vi "ROI entry screen-Fit and sanity check ROIs.vi"(10 "Old ROI file's data in":dbl[][](array[numeric])=[[0.0, 0.0, 0.0, 888.0, 200.0, 60.0, 888.0, 0.0, 0.0], [0.0, 0.0, 0.0, 888.0, 250.0, 70.0, 888.0, 50.0, 10.0], [0.0, 0.0, 0.0, 0.0, 80.0, 250.0, 888.0, 20.0, 50.0]] format="%#_6f", 11 "ROI fit info":T1 {"ROI fit info"."Frame size"."Old" items=["100X100"=100, "128X128"=128, "200X200"=200, "256X256"=256, "512X512"=512, "1024x1024"=1024, "2048x2048"=2048]; "ROI fit info"."Frame size"."New" items=["100X100"=100, "128X128"=128, "200X200"=200, "256X256"=256, "512X512"=512, "1024x1024"=1024, "2048x2048"=2048]}) -> (2 "Fitted ROI data":dbl[][](array[numeric]) format="%#_6f")   [LabVIEW 2020]
uses:
  Typedefs/ROI fitting info cluster.ctl
  Typedefs/Frame Size.ctl
panel:
  out "Mismatch":bool
  out "Vertical?":bool[](array[boolean])
  out "Output OK (mismatch fixed)":bool
  # "NOTE:\nThe default values saved in the controls are used to demonstrate how a rounding error in the conversion of the second ROI is corrected by the \"Check & Correct\" module."
  # "X start"
  # "Y start"
  # "X stop"
  # "Y stop"
  # "X start"
  # "Y start"
  # "X stop"
  # "Y stop"
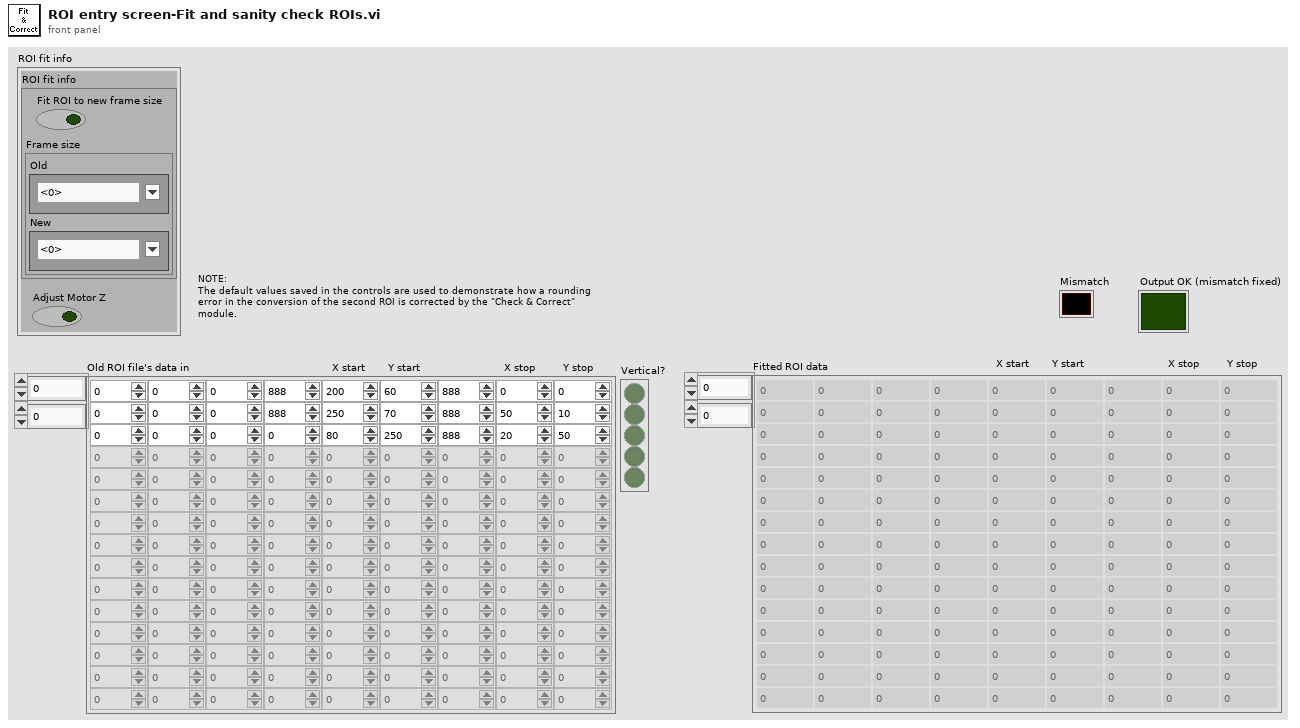
[diagram p1: front panel]
types:
  T1 = typedef "ROI fitting info cluster.ctl" = cluster{"ROI fit info":cluster{"Fit ROI to new frame size":bool, "Frame size":cluster{"Old":T2, "New":T2}}, "Adjust Motor Z":bool}
  T2 = typedef "Frame Size.ctl" = u16
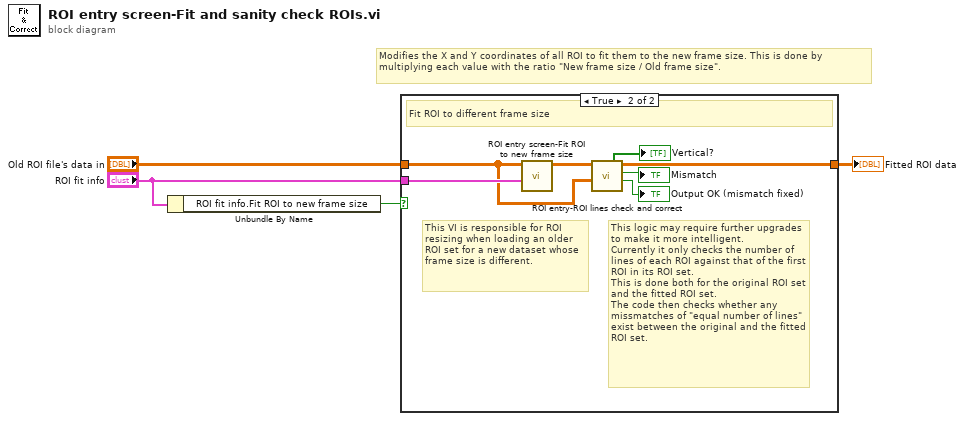
[diagram p0: block diagram]
diagram:
  # "Modifies the X and Y coordinates of all ROI to fit them to the new frame size. This is done by multiplying each value with the ratio \"New frame size / Old frame size\"."
  n1 = Unbundle By Name("ROI fit info") -> ("ROI fit info.Fit ROI to new frame size"=w4:bool)
  n2 = case shown="True" w4 {
    tunnel: "Old ROI file's data in" -> [w5 w7]
    tunnel: [w5 w11] -> w3
    tunnel: "ROI fit info" -> [_ w8]
    frame False {
      # "No need to adjust the ROI set"
    }
    frame True {
      # "This VI is responsible for ROI resizing when loading an older ROI set for a new dataset whose frame size is different."
      # "This logic may require further upgrades to make it more intelligent.\nCurrently it only checks the number of lines of each ROI against that of the first ROI in its ROI set.\nThis is done both for the original ROI set and the fitted ROI set.\nThe code then checks whether any missmatches of \"equal number of lines\" exist between the original and the fitted ROI set."
      # "Fit ROI to different frame size"
      n3 = call "ROI entry screen-Fit ROI to new frame size.vi"("ROI fit info"=w8, "Old ROI file's data in"=w7) -> ("Old ROI file's data out"=w6:dbl[][])  [unwired: 9 in]
      n4 = call "ROI entry-ROI lines check and correct.vi"("Old ROI file's data in"=w7, "New ROI file's data in in"=w6) -> ("Final OK"=→"Output OK (mismatch fixed)":bool, "Mismatch"=→"Mismatch":bool, "New ROI file's data out"=w11:dbl[][], "Vertical?"=→"Vertical?":bool[])  [unwired: 6 in]
    }
  }
  "Fitted ROI data" <- w3
